vi "Has Recievers.vi"(8 "error in (no error)":errorcluster, 11 "Pub Sub Message Channel in":refnum<class "Pub Sub Message Channel.lvclass">) -> (0 "error out":errorcluster, 2 "Has Recievers":bool, 3 "Pub Sub Message Channel out":refnum<class "Pub Sub Message Channel.lvclass">)   [LabVIEW 2020, in "Actor Pub Sub Channels.lvlib" / "Pub Sub Message Channel.lvclass"]
uses:
  Pub Sub Message Channel.lvclass
  Pub Sub Message Channel.lvclass/Pub Sub Message Channel.ctl
  <vilib>/ActorFramework/Message Enqueuer/Message Enqueuer.lvclass
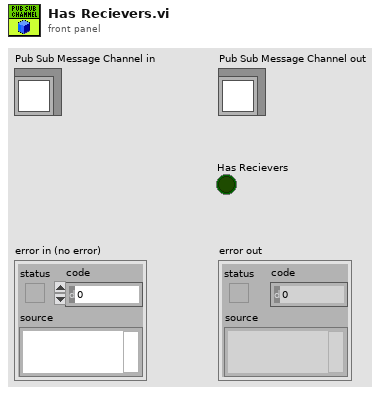
[diagram p1: front panel]
types:
  T1 = map{refnum<class "Message Enqueuer.lvclass">, string}
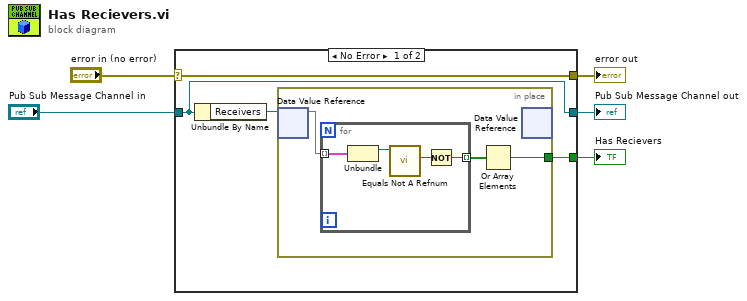
[diagram p0: block diagram]
diagram:
  n1 = case shown="No Error" "error in (no error)" {
    selector: "error in (no error)" -> [w9 w18]
    tunnel: [w9 w18] -> w4
    tunnel: [w8 w17] -> w2
    tunnel: "Pub Sub Message Channel in" -> [w8 w17]
    tunnel: [w6 _] -> w1
    frame No Error {
      n2 = Unbundle By Name(w8) -> ("Receivers"=w7:refnum<data-value>)
      n3 = in-place {
        in-place-border: [w10] -> w6
        n4 = in-place-dvr #1(w7) -> (w12:T1)  [unwired: 1 out]
        n5 = for {
          tunnel: w12 -> [w16] mode=indexing
          tunnel: [w13] -> w11 mode=indexing
          n6 = Unbundle(w16) -> ("Message Enqueuer"=w15:refnum<class "Message Enqueuer.lvclass">)  [unwired: 1 out]
          n7 = call <vilib>:"Equals Not A Refnum.vi"("Message Enqueuer"=w15) -> ("Not a refnum?"=w14:bool)  [unwired: 10 in]
          n8 = Not(x=w14) -> (.not. x?=w13:bool)
        }
        n9 = Or Array Elements(Boolean array=w11) -> (logical OR=w10:bool)
        n10 = in-place-dvr #1() -> ()  [unwired: 1 in, 2 out]
      }
    }
    frame Error {
    }
  }
  "error out" <- w4
  "Pub Sub Message Channel out" <- w2
  "Has Recievers" <- w1
